vi "check_addtional_soft_limits.vi"(8 "error in (no error)":errorcluster caption="错误输入（无错误）", 10 "pos":dbl[](array[numeric]), 11 "MotorSystem 输入":refnum<class "MotorSystem.lvclass">) -> (0 "error out":errorcluster caption="错误输出", 2 "out of limits?":bool, 3 "MotorSystem 输出":refnum<class "MotorSystem.lvclass">)   [LabVIEW 2016, in "MotionControl_UFO_3DOF.lvlib" / "MotorSystem.lvclass"]
uses:
  <userlib>/MotionControl_UFO_3DOF/MotorSystem/MotorSystem.lvclass
  <userlib>/MotionControl_UFO_3DOF/MotorSystem/MotorSystem.lvclass/MotorSystem.ctl
panel:
  # "(dims mismatch? == false && out of limits? == true) out of limits\notherwise ignore"
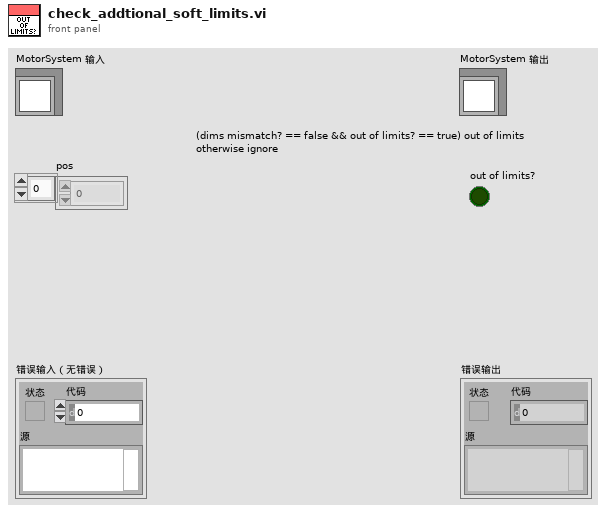
[diagram p1: front panel]
types:
  T1 = cluster{"array for a soft limit":cluster{"dim name":string, "soft limit":cluster{"min":dbl, "max":dbl}}[]}[]
  T2 = cluster{"dim name":string, "soft limit":cluster{"min":dbl, "max":dbl}}[]
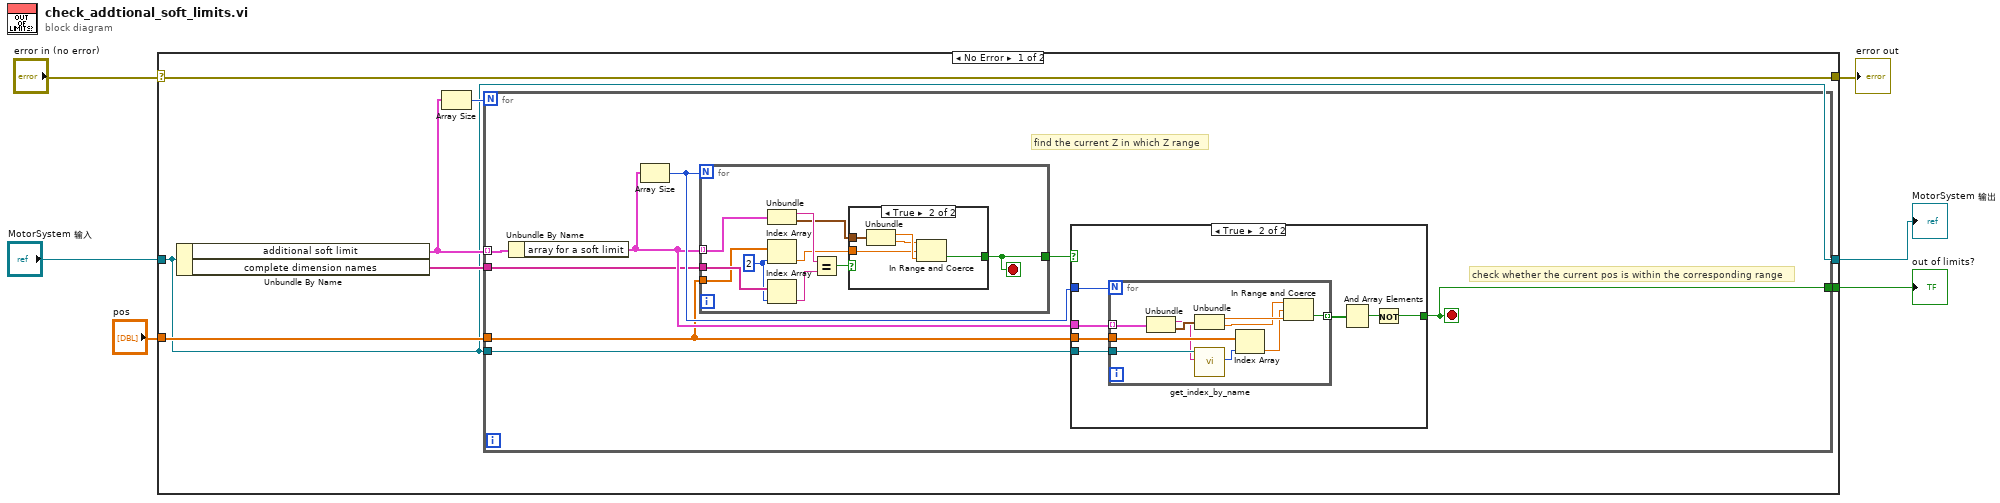
[diagram p0: block diagram]
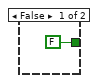
[diagram p3: hidden frame]
diagram:
  n1 = case shown="No Error" "error in (no error)" {
    selector: "error in (no error)" -> [w13 w57]
    tunnel: [w13 w57] -> w5
    tunnel: [w7 w56] -> w3
    tunnel: "MotorSystem 输入" -> [w7 w56]
    tunnel: "pos" -> [w10 _]
    tunnel: [w8 _] -> w1
    frame No Error {
      n2 = Unbundle By Name(w7) -> ("additional soft limit"=w11:T1, "complete dimension names"=w9:string[])
      n3 = Array Size(array=w11) -> (size(s)=w12:i32)
      n4 = for {
        N: w12 -> [_]
        tunnel: w11 -> [w21] mode=indexing
        tunnel: w10 -> [w16]
        tunnel: w9 -> [w17]
        tunnel: [w15] -> w8
        tunnel: w7 -> [w14]
        stop <- w15 stop-if-true
        # "check whether the current pos is within the corresponding range"
        # "find the current Z in which Z range"
        n5 = Unbundle By Name(w21) -> ("array for a soft limit"=w18:T2)
        n6 = Array Size(array=w18) -> (size(s)=w19:i32)
        n7 = for {
          N: w19 -> [_]
          tunnel: w18 -> [w49] mode=indexing
          tunnel: w16 -> [w46]
          tunnel: w17 -> [w47]
          tunnel: [w40] -> w20
          stop <- w40 stop-if-true
          w45 = 2 ("索引")
          n8 = Unbundle(w49) -> ("dim name"=w48:string, "soft limit"=w42:cluster{"min":dbl, "max":dbl})
          n9 = Index Array(array=w46, index=w45) -> (element=w41:dbl)
          n10 = Index Array(array=w47, index=w45) -> (element=w44:string)
          n11 = Equal?(x=w48, y=w44) -> (x = y?=w43:bool)
          n12 = case shown="True" w43 {
            tunnel: w42 -> [_ w55]
            tunnel: w41 -> [_ w52]
            tunnel: [FALSE w51] -> w40
            frame False {
            }
            frame True {
              n13 = Unbundle(w55) -> ("min"=w54:dbl, "max"=w53:dbl)
              n14 = In Range and Coerce(upper limit=w53, x=w52, lower limit=w54) -> (In Range?=w51:bool)  [unwired: 1 out]
            }
          }
        }
        n15 = case shown="True" w20 {
          selector: w20 -> [w22 _]
          tunnel: w19 -> [_ w29]
          tunnel: w18 -> [_ w28]
          tunnel: w16 -> [_ w27]
          tunnel: [w22 w24] -> w15
          tunnel: w14 -> [_ w23]
          frame False {
          }
          frame True {
            n16 = for {
              N: w29 -> [_]
              tunnel: w28 -> [w39] mode=indexing
              tunnel: w27 -> [w38]
              tunnel: [w33] -> w26 mode=indexing
              tunnel: w23 -> [w32]
              n17 = Unbundle(w39) -> ("dim name"=w31:string, "soft limit"=w37:cluster{"min":dbl, "max":dbl})
              n18 = Unbundle(w37) -> ("min"=w36:dbl, "max"=w35:dbl)
              n19 = call <userlib>:"get_index_by_name.vi"("name"=w31, "MotorSystem 输入"=w32) -> ("index (0-based)"=w30:u32)  [unwired: 7 in, 2 out]
              n20 = Index Array(array=w38, index=w30) -> (element=w34:dbl)
              n21 = In Range and Coerce(upper limit=w35, x=w34, lower limit=w36) -> (In Range?=w33:bool)  [unwired: 1 out]
            }
            n22 = And Array Elements(Boolean array=w26) -> (logical AND=w25:bool)
            n23 = Not(x=w25) -> (.not. x?=w24:bool)
          }
        }
      }
    }
    frame Error {
    }
  }
  "error out" <- w5
  "MotorSystem 输出" <- w3
  "out of limits?" <- w1
